vi "Model 3566-Buzzer.vi"(8 "error in":errorcluster, 9 "Sound Volume":T2(ring), 10 "Command":T3(ring), 11 "Model 3566 Setting In":T1) -> (0 "error out":errorcluster, 2 "Respond":string, 3 "Model 3566 Setting Out":T1)   [LabVIEW 2018]
uses:
  Data Def/Model 3566-Setting.ctl
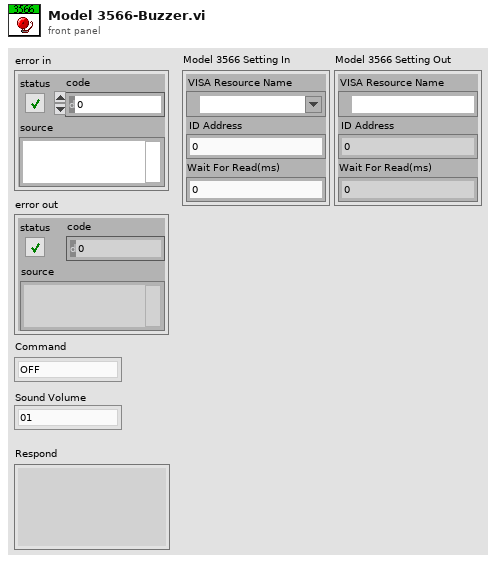
[diagram p1: front panel]
types:
  T1 = typedef "Model 3566-Setting.ctl" = cluster{"VISA Resource Name":refnum<visa-resource-name>, "ID Address":u8, "Wait For Read(ms)":u32}
  T2 = enum16{"01", "02", "03", "04", "05", "06", "07", "08", "09", "10"}
  T3 = enum16{"OFF", "GO", "HI", "LO", "HILO", "PASS", "FAIL", "GOOD", "NG"}
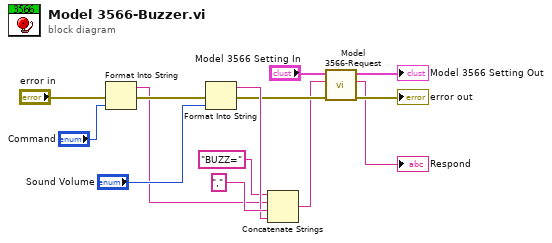
[diagram p0: block diagram]
diagram:
  n1 = Format Into String(error in="error in", "Command") -> (resulting string=w4:string, error out=w7:errorcluster)  [unwired: 2 in]
  n2 = Format Into String(error in=w7, "Sound Volume") -> (resulting string=w13:string, error out=w10:errorcluster)  [unwired: 2 in]
  n3 = Concatenate Strings("BUZZ=" ("string"), w4, "," ("string"), w13) -> (w9:string)
  n4 = call "Model 3566-Request.vi"("error in"=w10, "Command"=w9, "Model 3566 Setting In"="Model 3566 Setting In") -> ("error out"=→"error out":errorcluster, "Respond"=→"Respond":string, "Model 3566 Setting Out"=→"Model 3566 Setting Out":T1)  [unwired: 6 in]
